vi "LSMcontroller_v66_improvedwfhandling.vi"() -> ()   [LabVIEW 2015] (continued)
                          frame False {
                          }
                          frame True {
                            n96 = call "createdatafolder.vi"("timestamp in"=w2289) -> ("current data path"=w2290:path, "timestamp out"=w2288:timestamp)
                            n97 = local write "data dir"(w2290) -> ()
                          }
                        }
                        n98 = stacked-sequence {
                          tunnel: w2285 -> [_ w2297 _ _ _ _ _ _ _ _]
                          tunnel: [_ _ _ _ _ w2440 _ _ _ _] -> w2283
                          tunnel: [_ _ _ _ _ w2439 _ _ _ _] -> w2282
                          tunnel: [_ _ _ _ _ w2438 _ _ _ _] -> w2281
                          tunnel: [_ _ _ _ _ w2437 _ _ _ _] -> w2280
                          tunnel: [_ _ _ _ _ w2436 _ _ _ _] -> w2279
                          tunnel: [_ _ _ _ _ w2435 _ _ _ _] -> w2278
                          tunnel: [_ _ _ _ _ w2434 _ _ _ _] -> w2277
                          tunnel: [_ _ _ _ _ w2433 _ _ _ _] -> w2276
                          tunnel: [_ _ _ _ _ w2432 _ _ _ _] -> w2275
                          tunnel: [_ _ _ _ _ w2431 _ _ _ _] -> w2274
                          tunnel: [_ _ _ _ _ w2430 _ _ _ _] -> w2273
                          tunnel: [_ _ _ _ _ w2429 _ _ _ _] -> w2272
                          tunnel: [_ _ _ _ _ w2428 _ _ _ _] -> w2271
                          tunnel: [_ _ _ _ _ w2427 _ _ _ _] -> w2270
                          frame #0 {
                            n99 = local read "AI channels"() -> (w2296:i32[])
                            n100 = local read "CI channels"() -> (w2295:i32[])
                            n101 = call "2pparameters.vi"("command"="get") -> ("params out"=w2293:T10)  [unwired: 1 in]
                            n102 = Bundle By Name(cluster=w2293, "aAI"=w2296, "aCI"=w2295) -> (w2294:T10)
                            n103 = call "2pparameters.vi"("Params in"=w2294, "command"="set") -> ()  [unwired: 1 out]
                          }
                          frame #1 {
                            n104 = local read "Vy-min ref"() -> (w2301:dbl)
                            n105 = local read "Vy-max ref"() -> (w2302:dbl)
                            n106 = local read "Angle ref"() -> (w2300:dbl)
                            n107 = local read "Vx-min ref"() -> (w2303:dbl)
                            n108 = local write "counts"(0 ("counts")) -> ()
                            n109 = local write "graphtab"(T5."image" ("graphtab")) -> ()
                            n110 = local read "Vx-max ref"() -> (w2304:dbl)
                            n111 = property on="Stop" class="Bool (strict)"("Visible"=TRUE, "DisabledEnum"=T7."Enabled" ("Disabled")) -> ()  [unwired: 2 in, 2 out]
                            n112 = property on="Start" class="Bool (strict)"("Visible"=FALSE, "DisabledEnum"=T7."Disabled and Grayed Out" ("Disabled")) -> ()  [unwired: 2 in, 2 out]
                            n113 = script code="Xic=(ximax+ximin)./2;\nYic=(yimax+yimin)./2;\nximin=ximin-Xic;\nymin=ymin-Yic;\nxirmin=ximin.*cos(pi/180.*phi)+yimin.*sin(pi./180.*phi)+Xic;\nyirmin=-ximin.*sin(pi./180.*phi)+yimin.*cos(pi./180.*phi)+Yic;"("ximax"=w2304, "ximin"=w2303, "yimax"=w2302, "yimin"=w2301, "phi"=w2300) -> ("xirmin"=w2299:dbl, "yirmin"=w2298:dbl)  [unwired: 1 in, 1 out]
                            n114 = stacked-sequence {
                              tunnel: w2297 -> [_ w2329 _]
                              frame #0 {
                                n115 = local read "Measurement"() -> (w2311:T4)
                                n116 = case shown="\"X-Y-Z stack\"" w2311 {
                                frame "X-Y-t movie", Default {
                                n117 = call "2pparameters.vi"("command"="get") -> ("params out"=w2314:T10)  [unwired: 1 in]
                                n118 = Bundle By Name(cluster=w2314, "type"="X-Y-t movie") -> (w2312:T10)
                                n119 = call "2pparameters.vi"("Params in"=w2312, "command"="set") -> ()  [unwired: 1 out]
                                }
                                frame "X-Y-Z stack" {
                                n120 = call "2pparameters.vi"("command"="get") -> ("params out"=w2319:T10)  [unwired: 1 in]
                                n121 = Bundle By Name(cluster=w2319, "type"="X-Y-Z stack") -> (w2317:T10)
                                n122 = call "2pparameters.vi"("Params in"=w2317, "command"="set") -> ()  [unwired: 1 out]
                                }
                                frame "Lifetime (scan)" {
                                n123 = call "2pparameters.vi"("command"="get") -> ("params out"=w2324:T10)  [unwired: 1 in]
                                n124 = Bundle By Name(cluster=w2324, "type"="Lifetime (scan)") -> (w2322:T10)
                                n125 = call "2pparameters.vi"("Params in"=w2322, "command"="set") -> ()  [unwired: 1 out]
                                }
                                }
                              }
                              frame #1 {
                                n126 = Format Date/Time String(time format string (%c)="%Y%m%d", seconds (now)=w2329) -> (date/time string=w2328:string)  [unwired: 1 in]
                                n127 = Format Date/Time String(time format string (%c)="%H%M%S", seconds (now)=w2329) -> (date/time string=w2327:string)  [unwired: 1 in]
                                n128 = call "2pparameters.vi"("command"="get") -> ("params out"=w2333:T10)  [unwired: 1 in]
                                n129 = Bundle By Name(cluster=w2333, "date"=w2328, "time"=w2327) -> (w2332:T10)
                                n130 = call "2pparameters.vi"("Params in"=w2332, "command"="set") -> ()  [unwired: 1 out]
                              }
                              frame #2 {
                                n131 = call "configuration.vi"("command"="get") -> ("config out"=w2343:T11)  [unwired: 2 in, 1 out]
                                n132 = Unbundle By Name(w2343) -> ("CI names"=w2344:string[], "AI names"=w2345:string[])
                                n133 = call "2pparameters.vi"("command"="get") -> ("params out"=w2339:T10)  [unwired: 1 in]
                                n134 = Unbundle By Name(w2339) -> ("aCI"=w2340:i32[], "aAI"=w2341:i32[])
                                n135 = for {
                                tunnel: w2340 -> [w2355] mode=indexing
                                tunnel: w2344 -> [w2356]
                                tunnel: [w2354] -> w2346 mode=indexing
                                n136 = Index Array(array=w2356, index=w2355) -> (element=w2354:string)
                                }
                                n137 = for {
                                tunnel: w2341 -> [w2352] mode=indexing
                                tunnel: w2345 -> [w2353]
                                tunnel: [w2351] -> w2347 mode=indexing
                                n138 = Index Array(array=w2353, index=w2352) -> (element=w2351:string)
                                }
                                n139 = Build Array (concatenate)(w2346, w2347) -> (w2337:string[])
                                n140 = for {
                                tunnel: w2337 -> [w2349] mode=indexing
                                tunnel: [w2348] -> w2336 mode=indexing
                                i -> [w2350]
                                n141 = Bundle("String"=w2349, w2350) -> (w2348:cluster{"String":string, i32})  [unwired: 1 in]
                                }
                                n142 = property on="image1list" class="Ring (strict)"("StringsAndValues[]"=w2336) -> ()  [unwired: 2 in, 2 out]
                                n143 = property on="image2list" class="Ring (strict)"("StringsAndValues[]"=w2336) -> ()  [unwired: 2 in, 2 out]
                              }
                            }
                            n144 = call "setposition.vi"("Vy"=w2298, "Vx"=w2299) -> ()  [unwired: 1 in]
                          }
                          frame #2 {
                            n145 = call "X-array-databuffer.vi"("command"=enum16{"get", "set", "clear", "append"}."clear") -> ()  [unwired: 3 in, 2 out]
                            n146 = call "Y-array-databuffer.vi"("command"=enum16{"get", "set", "clear", "append"}."clear") -> ()  [unwired: 3 in, 2 out]
                            n147 = call "2pparameters.vi"("command"="get") -> ("params out"=w2359:T10)  [unwired: 1 in]
                            n148 = Unbundle By Name(w2359) -> ("autoshutter"=w2360:bool, "auto OD"=w2357:bool)
                            n149 = call "allAI-temp_img.vi"("command"=enum16{"get", "set", "clear", "append"}."clear") -> ()  [unwired: 3 in, 2 out]
                            n150 = case shown="True" w2357 {
                              frame False {
                              }
                              frame True {
                                n151 = call "configuration.vi"("command"="get") -> ("config out"=w2368:T11)  [unwired: 2 in, 1 out]
                                n152 = Unbundle By Name(w2368) -> ("image OD"=w2369:u16)
                                n153 = local read "ODfilt"() -> (w2366:u16)
                                n154 = call "filterwheelcontrol_nothorlabslib.vi"("Current OD filt"=w2366, "New ODfilt"=w2369) -> ()  [unwired: 1 in]
                              }
                            }
                            n155 = case shown="True" w2360 {
                              frame False {
                              }
                              frame True {
                                n156 = call "shuttercontrol.vi"("command"="close") -> ()  [unwired: 1 in, 1 out]
                              }
                            }
                            n157 = call "CH1-temp.vi"("command"=enum16{"get", "set", "clear", "add row"}."clear") -> ()  [unwired: 3 in, 2 out]
                            n158 = call "CH2-temp.vi"("command"=enum16{"get", "set", "clear", "add row"}."clear") -> ()  [unwired: 3 in, 2 out]
                          }
                          frame #3 {
                            n159 = local read "avpp"() -> (w2403:i32)
                            n160 = local read "Angle ref"() -> (w2402:dbl)
                            n161 = local read "ROI Type"() -> (w2401:u16)
                            n162 = local read "xpixels ref"() -> (w2398:i32)
                            n163 = local read "Vx-min ref"() -> (w2397:dbl)
                            n164 = local read "Vx-max ref"() -> (w2396:dbl)
                            n165 = local read "ypixels ref"() -> (w2394:i32)
                            n166 = local read "Vy-min ref"() -> (w2395:dbl)
                            n167 = local read "Vy-max ref"() -> (w2391:dbl)
                            n168 = local read "Sampling rate"() -> (w2385:dbl)
                            n169 = local read "finite samples"() -> (w2386:bool)
                            n170 = local read "continuous"() -> (w2389:bool)
                            n171 = local read "wavdet"() -> (w2390:bool)
                            n172 = local read "# of frames"() -> (w2388:i32)
                            n173 = local read "maxbufferAI"() -> (w2387:i32)
                            n174 = local read "Override AI buffer"() -> (w2371:bool)
                            n175 = call "2pparameters.vi"("command"="get") -> ("params out"=w2400:T10)  [unwired: 1 in]
                            n176 = Bundle By Name(cluster=w2400, "avpp"=w2403, "Angle Img"=w2402, "Xpixels Img"=w2398, "Vx-min Img"=w2397, "VX-max Img"=w2396, "Ypixels Img"=w2394, "Vy-min Img"=w2395, "Vy-max Img"=w2391, "srate"=w2385, "srate Img"=w2385, "finite"=w2386, "cont"=w2389, "wavdet"=w2390, "measpoints"=w2388, "maxbufferAI"=w2387, "Drawing Mode"=w2401, "Vz-reset"=0.0, "AIoverride"=w2371) -> (w2392:T10)
                            n177 = call "2pparameters.vi"("Params in"=w2392, "command"="set") -> ()  [unwired: 1 out]
                            n178 = local read "Vholding (mV)"() -> (w2374:sgl)
                            n179 = local read "Current Clamp"() -> (w2380:bool)
                            n180 = local read "Voltage Clamp"() -> (w2379:bool)
                            n181 = local read "OCgain"() -> (w2375:sgl)
                            n182 = local read "CC_ICgain"() -> (w2378:dbl)
                            n183 = local read "holdon"() -> (w2373:bool)
                            n184 = call "patchparameters.vi"("command"="get") -> ("Params out"=w2382:T13)  [unwired: 1 in]
                            n185 = Bundle By Name(cluster=w2382, "VC"=w2379, "CC"=w2380, "CC_icg (pA/mv)"=w2378, "VC_icg (mV/mV)"=sgl 10.0, "OCG (mV/pA)"=w2375, "OVG (mV/mV)"=0.1, "Vhold (mV)"=w2374, "holdon"=w2373) -> (w2381:T13)
                            n186 = call "patchparameters.vi"("Params in"=w2381, "command"="set") -> ()  [unwired: 1 out]
                          }
                          frame #4 {
                            # "Generate Waveforms for Scanning Mirrors"
                            n187 = call "2pparameters.vi"("command"="get") -> ("params out"=w2418:T10)  [unwired: 1 in]
                            n188 = Unbundle By Name(w2418) -> ("srate Img"=w2417:sgl, "Angle Img"=w2416:dbl, "VX-max Img"=w2415:dbl, "Vx-min Img"=w2414:dbl, "Xpixels Img"=w2413:i32, "Ypixels Img"=w2412:i32, "Vy-max Img"=w2411:dbl, "Vy-min Img"=w2410:dbl, "Drawing Mode"=w2409:u16)
                            n189 = call "ROI-databuffer.vi"("command"=enum16{"get", "set", "clear", "append"}."get") -> ("array out"=w2408:cluster{"x":sgl, "y":sgl}[])  [unwired: 4 in]
                            n190 = call "ScanningWaveform_v4.vi"("Vy-min"=w2410, "Vy-max"=w2411, "yPixels/tPixels"=w2412, "xPixels/rPixels"=w2413, "Vx-min"=w2414, "Vx-max"=w2415, "Drawing Mode"=w2409, "Angle"=w2416, "AOrate"=w2417, "Points"=w2408) -> ("numPixels"=w2404:dbl, "Y-WaveArray"=w2407:dbl[], "P"=w2405:dbl, "X-WaveArray"=w2406:dbl[])  [unwired: 6 in]
                            n191 = call "2pparameters.vi"("command"="get") -> ("params out"=w2426:T10)  [unwired: 1 in]
                            n192 = call "Y-array-databuffer.vi"("array in"=w2407, "command"=enum16{"get", "set", "clear", "append"}."set") -> ()  [unwired: 2 in, 2 out]
                            n193 = call "X-array-databuffer.vi"("array in"=w2406, "command"=enum16{"get", "set", "clear", "append"}."set") -> ()  [unwired: 2 in, 2 out]
                            n194 = Bundle By Name(cluster=w2426, "P"=w2405, "sAOxy"=w2404) -> (w2423:T10)
                            n195 = call "2pparameters.vi"("Params in"=w2423, "command"="set") -> ()  [unwired: 1 out]
                          }
                          frame #5 {
                            # "rem2Ps"
                            # "A2Ps"
                            # "Al"
                            # "Rl"
                            n196 = stacked-sequence {
                              seq-local: [w2445 _ _ _ _ _ _ _ _ _ _] -> [_ w2557 _ w2612 _ w2692 _ _ _ _ _]
                              seq-local: [w2446 _ _ _ _ _ _ _ _ _ _] -> [_ w2558 w2568 _ w2661 _ _ _ _ _ _]
                              seq-local: [_ _ w2567 _ _ _ _ _ _ _ _] -> [_ _ _ _ w2655 _ _ _ _ _ _]
                              seq-local: [_ _ _ w2611 _ _ _ _ _ _ _] -> [_ _ _ _ _ w2691 _ _ _ _ _]
                              seq-local: [w2442 _ _ _ _ _ _ _ _ _ _] -> [_ w2554 _ _ _ _ _ _ w2877 w2945 _]
                              seq-local: [w2441 _ _ _ _ _ _ _ _ _ _] -> [_ w2553 _ _ _ _ _ _ w2878 w2946 _]
                              seq-local: [w2448 _ _ _ _ _ _ _ _ _ _] -> [_ _ _ _ _ _ w2730 _ w2876 w2944 _]
                              seq-local: [w2444 _ _ _ _ _ _ _ _ _ _] -> [_ w2552 _ _ _ _ w2729 w2797 _ _ _]
                              seq-local: [w2443 _ _ _ _ _ _ _ _ _ _] -> [_ w2551 _ _ _ _ w2728 w2796 _ _ _]
                              seq-local: [w2447 _ _ _ _ _ _ _ _ _ _] -> [_ _ _ _ _ _ w2727 w2795 _ _ _]
                              tunnel: [_ _ w2566 _ _ _ _ _ _ _ _] -> w2439
                              tunnel: [_ _ w2565 _ _ _ _ _ _ _ _] -> w2438
                              tunnel: [w2446 _ _ _ _ _ _ _ _ _ _] -> w2440
                              tunnel: [w2445 _ _ _ _ _ _ _ _ _ _] -> w2437
                              tunnel: [_ _ _ w2610 _ _ _ _ _ _ _] -> w2436
                              tunnel: [_ _ _ w2609 _ _ _ _ _ _ _] -> w2435
                              tunnel: [w2444 _ _ _ _ _ _ _ _ _ _] -> w2434
                              tunnel: [w2443 _ _ _ _ _ _ _ _ _ _] -> w2433
                              tunnel: [_ _ _ _ _ _ w2726 _ _ _ _] -> w2432
                              tunnel: [_ _ _ _ _ _ _ w2794 _ _ _] -> w2431
                              tunnel: [w2442 _ _ _ _ _ _ _ _ _ _] -> w2430
                              tunnel: [w2441 _ _ _ _ _ _ _ _ _ _] -> w2429
                              tunnel: [_ _ _ _ _ _ _ _ w2875 _ _] -> w2428
                              tunnel: [_ _ _ _ _ _ _ _ _ w2943 _] -> w2427
                              frame #0 {
                                # "for a next version, give ome thought to\nthe possibilit of intermittently updating the\nwaveforms. it will have to be a calculation\nbased on speed of CPU and program on the one hand\nand length of measurement on the other. but then it should be possible, in principle, to \nupdate the waveform on the fly and that way cut up a longer measurement in smaller parts."
                                # "Y"
                                # "X"
                                n197 = stacked-sequence {
                                tunnel: [w2449 _ _ _] -> w2446
                                tunnel: [_ w2461 _ _] -> w2445
                                tunnel: [_ _ _ w2518] -> w2441
                                tunnel: [_ _ _ w2517] -> w2442
                                tunnel: [_ _ _ w2516] -> w2448
                                tunnel: [_ _ w2476 _] -> w2444
                                tunnel: [_ _ w2475 _] -> w2443
                                tunnel: [_ _ w2474 _] -> w2447
                                frame #0 {
                                n198 = call "configuration.vi"("command"="get") -> ("config out"=w2451:T11)  [unwired: 2 in, 1 out]
                                n199 = Unbundle By Name(w2451) -> ("Voltage to Xgalvo"=w2450:i32)
                                n200 = call "2pparameters.vi"("command"="get") -> ("params out"=w2455:T10)  [unwired: 1 in]
                                n201 = in-place {
                                in-place-border: w2450 -> [w2460]
                                in-place-border: [w2457] -> w2449
                                n202 = in-place-cluster #1(w2455) -> ("aAO"=w2459:u32[])
                                n203 = call "add channel to active arrayv2.vi"("line array in"=w2459, "line to add"=w2460) -> ("line array out"=w2458:u32[], "addition"=w2457:bool)  [unwired: 1 out]
                                n204 = in-place-cluster #1("aAO"=w2458) -> (w2453:T10)
                                }
                                n205 = call "2pparameters.vi"("Params in"=w2453, "command"="set") -> ()  [unwired: 1 out]
                                }
                                frame #1 {
                                n206 = call "configuration.vi"("command"="get") -> ("config out"=w2463:T11)  [unwired: 2 in, 1 out]
                                n207 = Unbundle By Name(w2463) -> ("Voltage to Ygalvo"=w2462:i32)
                                n208 = call "2pparameters.vi"("command"="get") -> ("params out"=w2467:T10)  [unwired: 1 in]
                                n209 = in-place {
                                in-place-border: w2462 -> [w2472]
                                in-place-border: [w2469] -> w2461
                                n210 = in-place-cluster #2(w2467) -> ("aAO"=w2471:u32[])
                                n211 = call "add channel to active arrayv2.vi"("line array in"=w2471, "line to add"=w2472) -> ("line array out"=w2470:u32[], "addition"=w2469:bool)  [unwired: 1 out]
                                n212 = in-place-cluster #2("aAO"=w2470) -> (w2465:T10)
                                }
                                n213 = call "2pparameters.vi"("Params in"=w2465, "command"="set") -> ()  [unwired: 1 out]
                                }
                                frame #2 {
                                n214 = call "2pparameters.vi"("command"="get") -> ("params out"=w2478:T10)  [unwired: 1 in]
                                n215 = Unbundle By Name(w2478) -> ("autoshutter"=w2477:bool, "wavdet"=w2473:bool)
                                n216 = case shown="True" w2477 {
                                tunnel: [w2483 w2503] -> w2476
                                tunnel: [w2482 FALSE ("removal")] -> w2475
                                tunnel: [w2481 w2501] -> w2474
                                tunnel: w2473 -> [w2480 _]
                                frame False {
                                n217 = case shown="False" w2480 {
                                tunnel: [FALSE ("addition") FALSE ("addition")] -> w2483
                                tunnel: [w2485 FALSE ("removal")] -> w2482
                                tunnel: [w2484 _] -> w2481
                                frame False {
                                n218 = call "configuration.vi"("command"="get") -> ("config out"=w2491:T11)  [unwired: 2 in, 1 out]
                                n219 = Unbundle By Name(w2491) -> ("2P shutter"=w2488:i32)
                                n220 = call "2pparameters.vi"("command"="get") -> ("params out"=w2489:T10)  [unwired: 1 in]
                                n221 = in-place {
                                in-place-border: w2488 -> [w2498]
                                in-place-border: [w2495] -> w2485
                                in-place-border: [w2494] -> w2484
                                n222 = in-place-cluster #3(w2489) -> ("aDO"=w2497:u32[])
                                n223 = call "remove channel from active arrayv2.vi"("line array in"=w2497, "line to remove"=w2498) -> ("line array out"=w2496:u32[], "removal"=w2495:bool, "index"=w2494:i32)
                                n224 = in-place-cluster #3("aDO"=w2496) -> (w2486:T10)
                                }
                                n225 = call "2pparameters.vi"("Params in"=w2486, "command"="set") -> ()  [unwired: 1 out]
                                }
                                frame True {
                                }
                                }
                                }
                                frame True {
                                n226 = call "configuration.vi"("command"="get") -> ("config out"=w2505:T11)  [unwired: 2 in, 1 out]
                                n227 = call "2pparameters.vi"("command"="get") -> ("params out"=w2509:T10)  [unwired: 1 in]
                                n228 = Unbundle By Name(w2505) -> ("2P shutter"=w2504:i32)
                                n229 = in-place {
                                in-place-border: w2504 -> [w2515]
                                in-place-border: [w2512] -> w2503
                                in-place-border: [w2511] -> w2501
                                n230 = in-place-cluster #4(w2509) -> ("aDO"=w2514:u32[])
                                n231 = call "add channel to active arrayv2.vi"("line array in"=w2514, "line to add"=w2515) -> ("line array out"=w2513:u32[], "addition"=w2512:bool, "index"=w2511:i32)
                                n232 = in-place-cluster #4("aDO"=w2513) -> (w2507:T10)
                                }
                                n233 = call "2pparameters.vi"("Params in"=w2507, "command"="set") -> ()  [unwired: 1 out]
                                }
                                }
                                }
                                frame #3 {
                                n234 = local read "Measurement"() -> (w2519:T4)
                                n235 = To Unsigned Long Integer(number=w2519) -> (unsigned 32bit integer=w2520:u32)
                                n236 = case shown="5..7" w2520 {
                                tunnel: [FALSE ("addition") w2538] -> w2518
                                tunnel: [w2523 FALSE ("removal")] -> w2517
                                tunnel: [w2521 w2536] -> w2516
                                frame 0..4, Default {
                                n237 = call "configuration.vi"("command"="get") -> ("config out"=w2529:T11)  [unwired: 2 in, 1 out]
                                n238 = Unbundle By Name(w2529) -> ("LT timestamp"=w2526:u32)
                                n239 = call "2pparameters.vi"("command"="get") -> ("params out"=w2527:T10)  [unwired: 1 in]
                                n240 = in-place {
                                in-place-border: w2526 -> [w2535]
                                in-place-border: [w2532] -> w2523
                                in-place-border: [w2531] -> w2521
                                n241 = in-place-cluster #5(w2527) -> ("aDO"=w2534:u32[])
                                n242 = call "remove channel from active arrayv2.vi"("line array in"=w2534, "line to remove"=w2535) -> ("line array out"=w2533:u32[], "removal"=w2532:bool, "index"=w2531:i32)
                                n243 = in-place-cluster #5("aDO"=w2533) -> (w2524:T10)
                                }
                                n244 = call "2pparameters.vi"("Params in"=w2524, "command"="set") -> ()  [unwired: 1 out]
                                }
                                frame 5..7 {
                                n245 = call "configuration.vi"("command"="get") -> ("config out"=w2544:T11)  [unwired: 2 in, 1 out]
                                n246 = Unbundle By Name(w2544) -> ("LT timestamp"=w2541:u32)
                                n247 = call "2pparameters.vi"("command"="get") -> ("params out"=w2542:T10)  [unwired: 1 in]
                                n248 = in-place {
                                in-place-border: w2541 -> [w2550]
                                in-place-border: [w2547] -> w2538
                                in-place-border: [w2546] -> w2536
                                n249 = in-place-cluster #6(w2542) -> ("aDO"=w2549:u32[])
                                n250 = call "add channel to active arrayv2.vi"("line array in"=w2549, "line to add"=w2550) -> ("line array out"=w2548:u32[], "addition"=w2547:bool, "index"=w2546:i32)
                                n251 = in-place-cluster #6("aDO"=w2548) -> (w2539:T10)
                                }
                                n252 = call "2pparameters.vi"("Params in"=w2539, "command"="set") -> ()  [unwired: 1 out]
                                }
                                }
                                }
                                }
                              }
                              frame #1 {
                                n253 = Or(x=w2557, y=w2558) -> (x .or. y?=w2556:bool)
                                n254 = case shown="True" w2556 {
                                frame False {
                                }
                                frame True {
                                # "update GUI"
                                n255 = call "Used AO lines.vi"() -> ("used AO names"=w2562:string[], "used AO lines"=w2564:tag[])  [unwired: 2 in]
                                n256 = control-ref of="Analog Lines Plot"() -> (w2563:refnum<vi>)
                                n257 = local write "Analog Used Lines"(w2564) -> ()
                                n258 = local write "Analog Used Names"(w2562) -> ()
                                n259 = call "prepAOWaveplot.vi"("WaveformGraph in"=w2563, "Analog Used Names"=w2562) -> ()  [unwired: 1 in]
                                }
                                }
                                n260 = Compound Arithmetic op=OR(w2554, w2553, w2552, w2551) -> (w2555:bool)
                                n261 = case shown="True" w2555 {
                                frame False {
                                }
                                frame True {
                                n262 = control-ref of="Digital Lines Plot"() -> (w2559:refnum<vi>)
                                n263 = call "Used DO lines.vi"() -> ("used DO names"=w2560:string[], "used DO lines"=w2561:tag[])  [unwired: 2 in]
                                n264 = local write "Digital Used Lines"(w2561) -> ()
                                n265 = local write "Digital Used Names"(w2560) -> ()
                                n266 = call "prepDOWaveplot.vi"("DigitalGraph in"=w2559, "used DO names"=w2560) -> ()  [unwired: 1 in]
                                }
                                }
                              }
                              frame #2 {
                                n267 = case shown="False" w2568 {
                                tunnel: [w2571 w2592] -> w2567
                                tunnel: [w2570 w2590] -> w2566
                                tunnel: [w2569 _] -> w2565
                                frame False {
                                n268 = stacked-sequence {
                                seq-local: [w2573 _] -> [_ w2586]
                                tunnel: [w2573 _] -> w2571
                                tunnel: [w2576 _] -> w2570
                                tunnel: [w2572 _] -> w2569
                                frame #0 {
                                n269 = call "configuration.vi"("command"="get") -> ("config out"=w2584:T11)  [unwired: 2 in, 1 out]
                                n270 = call "waveformparamsv2.vi"("command"="get") -> ("Params out"=w2578:T14)  [unwired: 4 in, 2 out]
                                n271 = Unbundle By Name(w2584) -> ("Voltage to Xgalvo"=w2585:i32)
                                n272 = call "2pparameters.vi"("command"="get") -> ("params out"=w2581:T10)  [unwired: 1 in]
                                n273 = Unbundle By Name(w2578) -> ("AO parameters"=w2577:T15)
                                n274 = Unbundle By Name(w2581) -> ("aAO"=w2582:u32[])
                                n275 = call "waveformsAObuffer.vi"("command"="get") -> ("AO wf out"=w2574:waveform(dbl)[])  [unwired: 1 in]
                                n276 = Search 1D Array(1D array=w2582, element=w2585) -> (index of element=w2573:i32)  [unwired: 1 in]
                                n277 = Index Array(array=w2574, index=w2573) -> (element=w2572:waveform(dbl))
                                n278 = Index Array(array=w2577, index=w2573) -> (element=w2576:T16)
                                }
                                frame #1 {
                                w2587 = 0.0 ("Step size (V)")
                                n279 = local read "Sampling rate"() -> (w2588:dbl)
                                n280 = call "replace AO XYwfparam.vi"("Baseline (V)"=w2587, "Start amplitude (V)"=w2587, "Cycles"=w2587, "Repeats"=w2587, "index of AO wave"=w2586, "Step size (V)"=w2587, "DC (%)"=w2587, "Sampling frequency (Hz)"=w2588, "Period (ms)"=w2587, "Cycle length (s)"=w2587, "Pulses"=w2587, "padding value"=w2587, "Matlab wave name"=path "xwave") -> ()  [unwired: 3 in]
                                }
                                }
                                }
                                frame True {
                                w2591 = 0.0 ("Repeats")
                                n281 = local read "Sampling rate"() -> (w2600:dbl)
                                n282 = call "2pparameters.vi"("command"="get") -> ("params out"=w2594:T10)  [unwired: 1 in]
                                n283 = call "configuration.vi"("command"="get") -> ("config out"=w2597:T11)  [unwired: 2 in, 1 out]
                                n284 = call "waveformparamsv2.vi"("command"="get") -> ("Params out"=w2606:T14)  [unwired: 4 in, 2 out]
                                n285 = Unbundle By Name(w2597) -> ("Voltage to Xgalvo"=w2598:i32)
                                n286 = Unbundle By Name(w2606) -> ("AO parameters"=w2603:T15)
                                n287 = Unbundle By Name(w2594) -> ("aAO"=w2595:u32[])
                                n288 = Search 1D Array(1D array=w2595, element=w2598) -> (index of element=w2592:i32)  [unwired: 1 in]
                                n289 = Index Array(array=w2603, index=0) -> (element=w2604:T16)
                                n290 = Bundle By Name(cluster=w2604, "AOtab"=-1.0 ("Repeats"), "Repeats"=w2591, "Cycles"=w2591, "Start amplitude (V)"=w2591, "Baseline (V)"=w2591, "Step size (V)"=w2591, "DC (%)"=w2591, "Sampling frequency (Hz)"=w2600, "Period (ms)"=w2591, "Offset (V)"=w2591, "Amplitude (V)"=w2591, "Frequency"=w2591, "Tri Repeats"=w2591, "phase shift (ms)"=w2591, "Pulses"=w2591, "Matlab wave file"=path "xwave", "padding value"=w2591) -> (w2590:T16)
                                n291 = Build Array(w2590) -> (w2601:T15)
                                n292 = call "waveformparamsv2.vi"("command"="add AO", "add AO"=w2601) -> ()  [unwired: 3 in, 3 out]
                                }
                                }
                              }
                              frame #3 {
                                n293 = case shown="False" w2612 {
                                tunnel: [w2615 w2636] -> w2611
                                tunnel: [w2614 w2634] -> w2610
                                tunnel: [w2613 _] -> w2609
                                frame False {
                                n294 = stacked-sequence {
                                seq-local: [w2617 _] -> [_ w2630]
                                tunnel: [w2617 _] -> w2615
                                tunnel: [w2620 _] -> w2614
                                tunnel: [w2616 _] -> w2613
                                frame #0 {
                                n295 = call "configuration.vi"("command"="get") -> ("config out"=w2628:T11)  [unwired: 2 in, 1 out]
                                n296 = call "waveformparamsv2.vi"("command"="get") -> ("Params out"=w2622:T14)  [unwired: 4 in, 2 out]
                                n297 = Unbundle By Name(w2628) -> ("Voltage to Ygalvo"=w2629:i32)
                                n298 = call "2pparameters.vi"("command"="get") -> ("params out"=w2625:T10)  [unwired: 1 in]
                                n299 = Unbundle By Name(w2622) -> ("AO parameters"=w2621:T15)
                                n300 = Unbundle By Name(w2625) -> ("aAO"=w2626:u32[])
                                n301 = call "waveformsAObuffer.vi"("command"="get") -> ("AO wf out"=w2618:waveform(dbl)[])  [unwired: 1 in]
                                n302 = Search 1D Array(1D array=w2626, element=w2629) -> (index of element=w2617:i32)  [unwired: 1 in]
                                n303 = Index Array(array=w2618, index=w2617) -> (element=w2616:waveform(dbl))
                                n304 = Index Array(array=w2621, index=w2617) -> (element=w2620:T16)
                                }
                                frame #1 {
                                w2631 = 0.0 ("Step size (V)")
                                n305 = local read "Sampling rate"() -> (w2632:dbl)
                                n306 = call "replace AO XYwfparam.vi"("Baseline (V)"=w2631, "Start amplitude (V)"=w2631, "Cycles"=w2631, "Repeats"=w2631, "index of AO wave"=w2630, "Step size (V)"=w2631, "DC (%)"=w2631, "Sampling frequency (Hz)"=w2632, "Period (ms)"=w2631, "Cycle length (s)"=w2631, "Pulses"=w2631, "padding value"=w2631, "Matlab wave name"=path "ywave") -> ()  [unwired: 3 in]
                                }
                                }
                                }
                                frame True {
                                w2635 = 0.0 ("Repeats")
                                n307 = local read "Sampling rate"() -> (w2645:dbl)
                                n308 = call "2pparameters.vi"("command"="get") -> ("params out"=w2638:T10)  [unwired: 1 in]
                                n309 = call "configuration.vi"("command"="get") -> ("config out"=w2641:T11)  [unwired: 2 in, 1 out]
                                n310 = call "waveformparamsv2.vi"("command"="get") -> ("Params out"=w2651:T14)  [unwired: 4 in, 2 out]
                                n311 = Unbundle By Name(w2641) -> ("Voltage to Ygalvo"=w2642:i32)
                                n312 = Unbundle By Name(w2651) -> ("AO parameters"=w2648:T15)
                                n313 = Unbundle By Name(w2638) -> ("aAO"=w2639:u32[])
                                n314 = Search 1D Array(1D array=w2639, element=w2642) -> (index of element=w2636:i32)  [unwired: 1 in]
                                n315 = Index Array(array=w2648, index=0) -> (element=w2649:T16)
                                n316 = Bundle By Name(cluster=w2649, "AOtab"=-1.0 ("Repeats"), "Repeats"=w2635, "Cycles"=w2635, "Start amplitude (V)"=w2635, "Baseline (V)"=w2635, "Step size (V)"=w2635, "DC (%)"=w2635, "Sampling frequency (Hz)"=w2645, "Period (ms)"=w2635, "Offset (V)"=w2635, "Amplitude (V)"=w2635, "Frequency"=w2635, "Tri Repeats"=w2635, "phase shift (ms)"=w2635, "Pulses"=w2635, "Matlab wave file"=path "ywave", "padding value"=w2635) -> (w2634:T16)
                                n317 = Build Array(w2634) -> (w2646:T15)
                                n318 = call "waveformparamsv2.vi"("command"="add AO", "add AO"=w2646) -> ()  [unwired: 3 in, 3 out]
                                }
                                }
                              }
                              frame #4 {
                                n319 = call "2pparameters.vi"("command"="get") -> ("params out"=w2658:T10)  [unwired: 1 in]
                                n320 = Unbundle By Name(w2658) -> ("wavdet"=w2657:bool, "sAOxy"=w2654:i32, "refwfsize"=w2653:dbl, "srate Img"=w2656:sgl)
                                n321 = case shown="False" w2657 {
                                tunnel: [w2662 w2672] -> w2660
                                tunnel: w2656 -> [w2663 w2674]
                                tunnel: w2654 -> [_ w2670]
                                tunnel: w2653 -> [_ w2669]
                                frame False {
                                n322 = call "X-array-databuffer.vi"("command"=enum16{"get", "set", "clear", "append"}."get") -> ("array out"=w2666:dbl[])  [unwired: 3 in, 1 out]
                                n323 = Reciprocal(x=w2663) -> (1/x=w2664:sgl)
                                n324 = Bundle By Name("Y"=w2666, "dt"=w2664) -> (w2662:waveform(dbl))  [unwired: 1 in]
                                }
                                frame True {
                                n325 = To Double Precision Float(number=w2670) -> (double precision float=w2671:dbl)
                                n326 = Divide(x=w2669, y=w2671) -> (x/y=w2667:dbl)
                                n327 = Round Toward +Infinity(x=w2667) -> (ceil(x): smallest int >= x=w2668:dbl)
                                n328 = call "X-array-databuffer.vi"("command"=enum16{"get", "set", "clear", "append"}."get") -> ("array out"=w2676:dbl[])  [unwired: 3 in, 1 out]
                                n329 = Reciprocal(x=w2674) -> (1/x=w2675:sgl)
                                n330 = for {
                                N: w2668 -> [_]
                                tunnel: w2676 -> [w2678]
                                tunnel: [w2678] -> w2673 mode=concatenating
                                }
                                n331 = Bundle By Name("Y"=w2673, "dt"=w2675) -> (w2672:waveform(dbl))  [unwired: 1 in]
                                }
                                }
                                n332 = case shown="False" w2661 {
                                tunnel: w2660 -> [w2680 w2686]
                                tunnel: w2655 -> [w2681 _]
                                frame False {
                                n333 = call "waveformsAObuffer.vi"("command"="get") -> ("AO wf out"=w2684:waveform(dbl)[])  [unwired: 1 in]
                                n334 = Replace Array Subset(array=w2684, new element=w2680, index=w2681) -> (w2679:waveform(dbl)[])
                                n335 = call "waveformsAObuffer.vi"("AO wf in"=w2679, "command"="set") -> ()  [unwired: 1 out]
                                }
                                frame True {
                                n336 = call "waveformsAObuffer.vi"("command"="get") -> ("AO wf out"=w2688:waveform(dbl)[])  [unwired: 1 in]
                                n337 = Build Array (concatenate)(w2688, w2686) -> (w2685:waveform(dbl)[])
                                n338 = call "waveformsAObuffer.vi"("AO wf in"=w2685, "command"="set") -> ()  [unwired: 1 out]
                                }
                                }
                              }
                              frame #5 {
                                n339 = call "2pparameters.vi"("command"="get") -> ("params out"=w2700:T10)  [unwired: 1 in]
                                n340 = Unbundle By Name(w2700) -> ("wavdet"=w2699:bool, "sAOxy"=w2697:i32, "refwfsize"=w2698:dbl, "srate Img"=w2693:sgl)
                                n341 = To Double Precision Float(number=w2697) -> (double precision float=w2696:dbl)
                                n342 = Divide(x=w2698, y=w2696) -> (x/y=w2695:dbl)
                                n343 = Round Toward +Infinity(x=w2695) -> (ceil(x): smallest int >= x=w2694:dbl)
                                n344 = case shown="True" w2699 {
                                tunnel: [w2704 w2709] -> w2690
                                tunnel: w2694 -> [_ w2713]
                                tunnel: w2693 -> [w2705 w2711]
                                frame False {
                                n345 = call "Y-array-databuffer.vi"("command"=enum16{"get", "set", "clear", "append"}."get") -> ("array out"=w2702:dbl[])  [unwired: 3 in, 1 out]
                                n346 = Reciprocal(x=w2705) -> (1/x=w2706:sgl)
                                n347 = Bundle By Name("Y"=w2702, "dt"=w2706) -> (w2704:waveform(dbl))  [unwired: 1 in]
                                }
                                frame True {
                                n348 = call "Y-array-databuffer.vi"("command"=enum16{"get", "set", "clear", "append"}."get") -> ("array out"=w2707:dbl[])  [unwired: 3 in, 1 out]
                                n349 = Reciprocal(x=w2711) -> (1/x=w2712:sgl)
                                n350 = for {
                                N: w2713 -> [_]
                                tunnel: w2707 -> [w2714]
                                tunnel: [w2714] -> w2710 mode=concatenating
                                }
                                n351 = Bundle By Name("Y"=w2710, "dt"=w2712) -> (w2709:waveform(dbl))  [unwired: 1 in]
                                }
                                }
                                n352 = case shown="False" w2692 {
                                tunnel: w2690 -> [w2717 w2722]
                                tunnel: w2691 -> [w2718 _]
                                frame False {
                                n353 = call "waveformsAObuffer.vi"("command"="get") -> ("AO wf out"=w2720:waveform(dbl)[])  [unwired: 1 in]
                                n354 = Replace Array Subset(array=w2720, new element=w2717, index=w2718) -> (w2715:waveform(dbl)[])
                                n355 = call "waveformsAObuffer.vi"("AO wf in"=w2715, "command"="set") -> ()  [unwired: 1 out]
                                }
                                frame True {
                                n356 = call "waveformsAObuffer.vi"("command"="get") -> ("AO wf out"=w2724:waveform(dbl)[])  [unwired: 1 in]
                                n357 = Build Array (concatenate)(w2724, w2722) -> (w2721:waveform(dbl)[])
                                n358 = call "waveformsAObuffer.vi"("AO wf in"=w2721, "command"="set") -> ()  [unwired: 1 out]
                                }
                                }
                              }
                              frame #6 {
                                n359 = Build Array(w2729, w2728) -> (w2732:bool[])
                                n360 = Boolean Array To Number(Boolean array=w2732) -> (number=w2731:u32)
                                n361 = case shown="0" w2731 {
                                tunnel: w2730 -> [_ _ _ _]
                                tunnel: w2727 -> [_ w2755 _ w2768]
                                tunnel: [_ w2754 _ w2765] -> w2726
                                frame 1 {
                                w2742 = 0.0 ("DOtab")
                                n362 = call "2pparameters.vi"("command"="get") -> ("params out"=w2739:T10)  [unwired: 1 in]
                                n363 = call "waveformparamsv2.vi"("command"="get") -> ("Params out"=w2750:T14)  [unwired: 4 in, 2 out]
                                n364 = Unbundle By Name(w2750) -> ("DO parameters"=w2748:T17)
                                n365 = Unbundle By Name(w2739) -> ("srate"=w2735:sgl, "sAOxy"=w2738:i32)
                                n366 = To Double Precision Float(number=w2735) -> (double precision float=w2733:dbl)
                                n367 = To Double Precision Float(number=w2735) -> (double precision float=w2734:dbl)
                                n368 = To Double Precision Float(number=w2738) -> (double precision float=w2737:dbl)
                                n369 = Divide(x=w2734, y=w2737) -> (x/y=w2736:dbl)
                                n370 = Index Array(array=w2748, index=0) -> (element=w2747:T18)
                                n371 = Bundle By Name(cluster=w2747, "Digital DC (%)"=100.0, "Digital phase"=w2742, "Digital Freq (Hz)"=w2736, "Sampling frequency (Hz)"=w2733, "Digital time offset (s)"=w2742, "padding value"=0.0, "matlab wave file"=path "2Pshutter", "DOtab"=0.0) -> (w2745:T18)
                                n372 = Build Array(w2745) -> (w2744:T17)
                                n373 = call "waveformparamsv2.vi"("command"="add DO", "add DO"=w2744) -> ()  [unwired: 3 in, 3 out]
                                }
                                frame 2 {
                                n374 = call "waveformparamsv2.vi"("command"="get") -> ("Params out"=w2757:T14)  [unwired: 4 in, 2 out]
                                n375 = in-place {
                                in-place-border: w2755 -> [w2761]
                                in-place-border: [w2760] -> w2754
                                n376 = in-place-cluster #7(w2757) -> ("DO parameters"=w2763:T17)
                                n377 = Delete From Array(array=w2763, length=1, index=w2761) -> (deleted portion=w2760:T17, array with subset deleted=w2762:T17)
                                n378 = in-place-cluster #7("DO parameters"=w2762) -> (w2756:T14)
                                }
                                n379 = call "waveformparamsv2.vi"("command"="set", "Params in"=w2756) -> ()  [unwired: 3 in, 3 out]
                                }
                                frame 3, Default {
                                }
                                frame 0 {
                                n380 = call "2pparameters.vi"("command"="get") -> ("params out"=w2770:T10)  [unwired: 1 in]
                                n381 = Unbundle By Name(w2770) -> ("wavdet"=w2767:bool, "autoshutter"=w2769:bool)
                                n382 = case shown="True" w2769 {
                                tunnel: w2768 -> [_ w2774]
                                tunnel: w2767 -> [_ w2773]
                                tunnel: [_ w2772] -> w2766
                                frame False {
                                }
                                frame True {
                                n383 = case shown="False" w2773 {
                                tunnel: w2774 -> [w2776 _]
                                tunnel: [w2775 _] -> w2772
                                frame False {
                                n384 = stacked-sequence {
                                tunnel: w2776 -> [w2778 w2792]
                                tunnel: [w2777 _] -> w2775
                                frame #0 {
                                n385 = call "waveformparamsv2.vi"("command"="get") -> ("Params out"=w2780:T14)  [unwired: 4 in, 2 out]
                                n386 = Unbundle By Name(w2780) -> ("DO parameters"=w2779:T17)
                                n387 = Index Array(array=w2779, index=w2778) -> (element=w2777:T18)
                                }
                                frame #1 {
                                w2791 = 0.0 ("padding value")
                                n388 = call "2pparameters.vi"("command"="get") -> ("params out"=w2789:T10)  [unwired: 1 in]
                                n389 = Unbundle By Name(w2789) -> ("srate"=w2786:sgl, "sAOxy"=w2788:i32)
                                n390 = To Double Precision Float(number=w2786) -> (double precision float=w2784:dbl)
                                n391 = To Double Precision Float(number=w2786) -> (double precision float=w2785:dbl)
                                n392 = To Double Precision Float(number=w2788) -> (double precision float=w2787:dbl)
                                n393 = Divide(x=w2785, y=w2787) -> (x/y=w2783:dbl)
                                n394 = call "replace DO wf param.vi"("Digital Freq (Hz)"=w2783, "Digital DC (%)"=100.0, "Digital phase"=w2791, "Sampling frequency (Hz)"=w2784, "Digital time offset (s)"=w2791, "index of DO wave"=w2792, "padding value"=w2791, "matlab wave file"=path "2Pshutter" ("matlab wave number")) -> ()  [unwired: 3 in]
                                }
                                }
                                }
                                frame True {
                                }
                                }
                                }
                                }
                                n395 = Build Array(w2766) -> (w2765:T17)
                                }
                                }
                              }
                              frame #7 {
                                n396 = Build Array(w2797, w2796) -> (w2799:bool[])
                                n397 = Boolean Array To Number(Boolean array=w2799) -> (number=w2798:u32)
                                n398 = case shown="2" w2798 {
                                tunnel: w2795 -> [_ w2841 _ w2848]
                                tunnel: [_ w2840 _ w2846] -> w2794
                                frame 1 {
                                n399 = call "2pparameters.vi"("command"="get") -> ("params out"=w2806:T10)  [unwired: 1 in]
                                n400 = Unbundle By Name(w2806) -> ("wavdet"=w2807:bool, "sAOxy"=w2809:i32, "refwfsize"=w2810:dbl, "srate Img"=w2808:sgl)
                                n401 = call "waveformsDObuffer.vi"("command"="get") -> ("DO wf out"=w2802:digitalwaveform[])  [unwired: 1 in]
                                n402 = case shown="False" w2807 {
                                tunnel: [w2815 w2825] -> w2804
                                tunnel: w2808 -> [w2820 w2836]
                                tunnel: w2809 -> [w2814 w2829]
                                tunnel: w2810 -> [_ w2833]
                                frame False {
                                w2818 = u16 0 items=["unsigned binary", "offset binary", "2's complement"] ("data format (offset binary)")
                                n403 = Initialize Array(sgl 1.0, w2814) -> (w2811:sgl[])
                                n404 = Reciprocal(x=w2820) -> (1/x=w2821:sgl)
                                n405 = Bundle By Name("Y"=w2811, "dt"=w2821) -> (w2816:waveform(sgl))  [unwired: 1 in]
                                n406 = call-poly <vilib>:"Analog to Digital.vi"("data format (offset binary)"=w2818, "compress digital (T)"=TRUE, "full-scale range (pk-pk)"=1.0, "resolution (16 bit)"=1, "analog waveform"=w2816) -> ("digital waveform"=w2815:digitalwaveform)  [unwired: 3 in, 3 out]
                                }
                                frame True {
                                w2828 = u16 0 items=["unsigned binary", "offset binary", "2's complement"] ("data format (offset binary)")
                                n407 = To Double Precision Float(number=w2829) -> (double precision float=w2834:dbl)
                                n408 = Initialize Array(sgl 1.0, w2829) -> (w2822:sgl[])
                                n409 = Divide(x=w2833, y=w2834) -> (x/y=w2831:dbl)
                                n410 = Round Toward +Infinity(x=w2831) -> (ceil(x): smallest int >= x=w2832:dbl)
                                n411 = for {
                                N: w2832 -> [_]
                                tunnel: w2822 -> [w2838]
                                tunnel: [w2838] -> w2835 mode=concatenating
                                }
                                n412 = Reciprocal(x=w2836) -> (1/x=w2837:sgl)
                                n413 = Bundle By Name("Y"=w2835, "dt"=w2837) -> (w2826:waveform(sgl))  [unwired: 1 in]
                                n414 = call-poly <vilib>:"Analog to Digital.vi"("data format (offset binary)"=w2828, "compress digital (T)"=TRUE, "full-scale range (pk-pk)"=1.0, "resolution (16 bit)"=1, "analog waveform"=w2826) -> ("digital waveform"=w2825:digitalwaveform)  [unwired: 3 in, 3 out]
                                }
                                }
                                n415 = Build Array (concatenate)(w2802, w2804) -> (w2800:digitalwaveform[])
                                n416 = call "waveformsDObuffer.vi"("DO wf in"=w2800, "command"="set") -> ()  [unwired: 1 out]
                                }
                                frame 2 {
                                n417 = call "waveformsDObuffer.vi"("command"="get") -> ("DO wf out"=w2843:digitalwaveform[])  [unwired: 1 in]
                                n418 = Delete From Array(array=w2843, length=1, index=w2841) -> (deleted portion=w2840:digitalwaveform[], array with subset deleted=w2839:digitalwaveform[])
                                n419 = call "waveformsDObuffer.vi"("DO wf in"=w2839, "command"="set") -> ()  [unwired: 1 out]
                                }
                                frame 3, Default {
                                }
                                frame 0 {
                                n420 = call "2pparameters.vi"("command"="get") -> ("params out"=w2850:T10)  [unwired: 1 in]
                                n421 = Unbundle By Name(w2850) -> ("autoshutter"=w2849:bool, "wavdet"=w2847:bool)
                                n422 = case shown="True" w2849 {
                                tunnel: w2848 -> [_ w2854]
                                tunnel: w2847 -> [_ w2853]
                                tunnel: [_ w2852] -> w2846
                                frame False {
                                }
                                frame True {
                                n423 = case shown="False" w2853 {
                                tunnel: w2854 -> [w2858 _]
                                tunnel: [w2856 _] -> w2852
                                frame False {
                                w2865 = u16 0 items=["unsigned binary", "offset binary", "2's complement"] ("data format (offset binary)")
                                n424 = call "2pparameters.vi"("command"="get") -> ("params out"=w2872:T10)  [unwired: 1 in]
                                n425 = Unbundle By Name(w2872) -> ("sAOxy"=w2874:i32, "srate Img"=w2873:sgl)
                                n426 = call "waveformsDObuffer.vi"("command"="get") -> ("DO wf out"=w2859:digitalwaveform[])  [unwired: 1 in]
                                n427 = Index Array(array=w2859, index=w2858) -> (element=w2857:digitalwaveform)
                                n428 = Build Array(w2857) -> (w2856:digitalwaveform[])
                                n429 = Initialize Array(sgl 1.0, w2874) -> (w2860:sgl[])
                                n430 = Reciprocal(x=w2873) -> (1/x=w2867:sgl)
                                n431 = Bundle By Name("Y"=w2860, "dt"=w2867) -> (w2863:waveform(sgl))  [unwired: 1 in]
                                n432 = call-poly <vilib>:"Analog to Digital.vi"("data format (offset binary)"=w2865, "compress digital (T)"=TRUE, "full-scale range (pk-pk)"=1.0, "resolution (16 bit)"=1, "analog waveform"=w2863) -> ("digital waveform"=w2870:digitalwaveform)  [unwired: 3 in, 3 out]
                                n433 = Replace Array Subset(array=w2859, new element=w2870, index=w2858) -> (w2855:digitalwaveform[])
                                n434 = call "waveformsDObuffer.vi"("DO wf in"=w2855, "command"="set") -> ()  [unwired: 1 out]
                                }
                                frame True {
                                }
                                }
                                }
                                }
                                }
                                }
                              }
                              frame #8 {
                                n435 = Build Array(w2878, w2877) -> (w2880:bool[])
                                n436 = Boolean Array To Number(Boolean array=w2880) -> (number=w2879:u32)
                                n437 = case shown="0" w2879 {
                                tunnel: w2876 -> [_ w2906 _ w2918]
                                tunnel: [_ w2905 _ w2916] -> w2875
                                frame 1 {
                                w2893 = 0.0 ("DOtab")
                                n438 = call "2pparameters.vi"("command"="get") -> ("params out"=w2891:T10)  [unwired: 1 in]
                                n439 = call "waveformparamsv2.vi"("command"="get") -> ("Params out"=w2901:T14)  [unwired: 4 in, 2 out]
                                n440 = Unbundle By Name(w2901) -> ("DO parameters"=w2899:T17)
                                n441 = Unbundle By Name(w2891) -> ("srate"=w2888:sgl, "sAOxy"=w2890:i32)
                                n442 = To Double Precision Float(number=w2888) -> (double precision float=w2886:dbl)
                                n443 = To Double Precision Float(number=w2888) -> (double precision float=w2887:dbl)
                                n444 = To Double Precision Float(number=w2890) -> (double precision float=w2882:dbl)
                                n445 = Divide(x=w2887, y=w2882) -> (x/y=w2889:dbl)
                                n446 = Index Array(array=w2899, index=0) -> (element=w2898:T18)
                                n447 = Divide(x=1.0 ("Digital DC (%)"), y=w2882) -> (x/y=w2884:dbl)
                                n448 = Multiply(x=100.0, y=w2884) -> (x*y=w2881:dbl)
                                n449 = Bundle By Name(cluster=w2898, "Digital DC (%)"=w2881, "Digital phase"=w2893, "Digital Freq (Hz)"=w2889, "Sampling frequency (Hz)"=w2886, "Digital time offset (s)"=w2893, "padding value"=0.0, "matlab wave file"=path "LT", "DOtab"=0.0) -> (w2896:T18)
                                n450 = Build Array(w2896) -> (w2895:T17)
                                n451 = call "waveformparamsv2.vi"("command"="add DO", "add DO"=w2895) -> ()  [unwired: 3 in, 3 out]
                                }
                                frame 2 {
                                n452 = call "waveformparamsv2.vi"("command"="get") -> ("Params out"=w2908:T14)  [unwired: 4 in, 2 out]
                                n453 = in-place {
                                in-place-border: w2906 -> [w2912]
                                in-place-border: [w2911] -> w2905
                                n454 = in-place-cluster #8(w2908) -> ("DO parameters"=w2914:T17)
                                n455 = Delete From Array(array=w2914, length=1, index=w2912) -> (deleted portion=w2911:T17, array with subset deleted=w2913:T17)
                                n456 = in-place-cluster #8("DO parameters"=w2913) -> (w2907:T14)
                                }
                                n457 = call "waveformparamsv2.vi"("command"="set", "Params in"=w2907) -> ()  [unwired: 3 in, 3 out]
                                }
                                frame 3, Default {
                                }
                                frame 0 {
                                n458 = local read "Measurement"() -> (w2920:T4)
                                n459 = To Unsigned Long Integer(number=w2920) -> (unsigned 32bit integer=w2919:u32)
                                n460 = case shown="5..7" w2919 {
                                tunnel: w2918 -> [_ w2922]
                                tunnel: [_ w2921] -> w2917
                                frame 0..4, Default {
                                }
                                frame 5..7 {
                                n461 = stacked-sequence {
                                tunnel: w2922 -> [w2924 w2933]
                                tunnel: [w2923 _] -> w2921
                                frame #0 {
                                n462 = call "waveformparamsv2.vi"("command"="get") -> ("Params out"=w2926:T14)  [unwired: 4 in, 2 out]
                                n463 = Unbundle By Name(w2926) -> ("DO parameters"=w2927:T17)
                                n464 = Index Array(array=w2927, index=w2924) -> (element=w2923:T18)
                                }
                                frame #1 {
                                w2941 = 0.0 ("padding value")
                                n465 = call "2pparameters.vi"("command"="get") -> ("params out"=w2939:T10)  [unwired: 1 in]
                                n466 = Unbundle By Name(w2939) -> ("srate"=w2937:sgl, "sAOxy"=w2938:i32)
                                n467 = To Double Precision Float(number=w2937) -> (double precision float=w2935:dbl)
                                n468 = To Double Precision Float(number=w2937) -> (double precision float=w2936:dbl)
                                n469 = To Double Precision Float(number=w2938) -> (double precision float=w2931:dbl)
                                n470 = Divide(x=1.0 ("Digital DC (%)"), y=w2931) -> (x/y=w2930:dbl)
                                n471 = Multiply(x=100.0, y=w2930) -> (x*y=w2929:dbl)
                                n472 = Divide(x=w2936, y=w2931) -> (x/y=w2934:dbl)
                                n473 = call "replace DO wf param.vi"("Digital Freq (Hz)"=w2934, "Digital DC (%)"=w2929, "Digital phase"=w2941, "Sampling frequency (Hz)"=w2935, "Digital time offset (s)"=w2941, "index of DO wave"=w2933, "padding value"=w2941, "matlab wave file"=path "LT" ("matlab wave number")) -> ()  [unwired: 3 in]
                                }
                                }
                                }
                                }
                                n474 = Build Array(w2917) -> (w2916:T17)
                                }
                                }
                              }
                              frame #9 {
                                n475 = Build Array(w2946, w2945) -> (w2948:bool[])
                                n476 = Boolean Array To Number(Boolean array=w2948) -> (number=w2947:u32)
                                n477 = case shown="2" w2947 {
                                tunnel: w2944 -> [_ w3000 _ w3004]
                                tunnel: [_ w2995 _ w3001] -> w2943
                                frame 1 {
                                n478 = call "2pparameters.vi"("command"="get") -> ("params out"=w2955:T10)  [unwired: 1 in]
                                n479 = Unbundle By Name(w2955) -> ("wavdet"=w2956:bool, "sAOxy"=w2958:i32, "refwfsize"=w2959:dbl, "srate Img"=w2957:sgl)
                                n480 = call "waveformsDObuffer.vi"("command"="get") -> ("DO wf out"=w2951:digitalwaveform[])  [unwired: 1 in]
                                n481 = case shown="True" w2956 {
                                tunnel: [w2963 w2976] -> w2953
                                tunnel: w2957 -> [w2972 w2991]
                                tunnel: w2958 -> [w2962 w2982]
                                tunnel: w2959 -> [_ w2988]
                                frame False {
